vi "simple_subscriber_try.vi"() -> ()   [LabVIEW 2014]
panel:
  out "JSON字符串 2":string
  in  "停止":bool
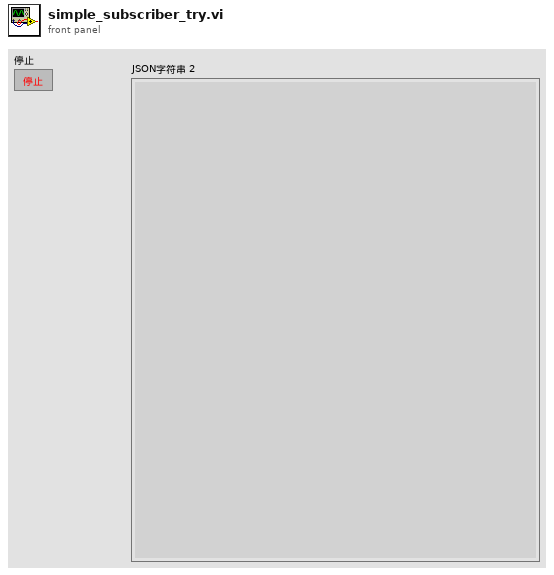
[diagram p1: front panel]
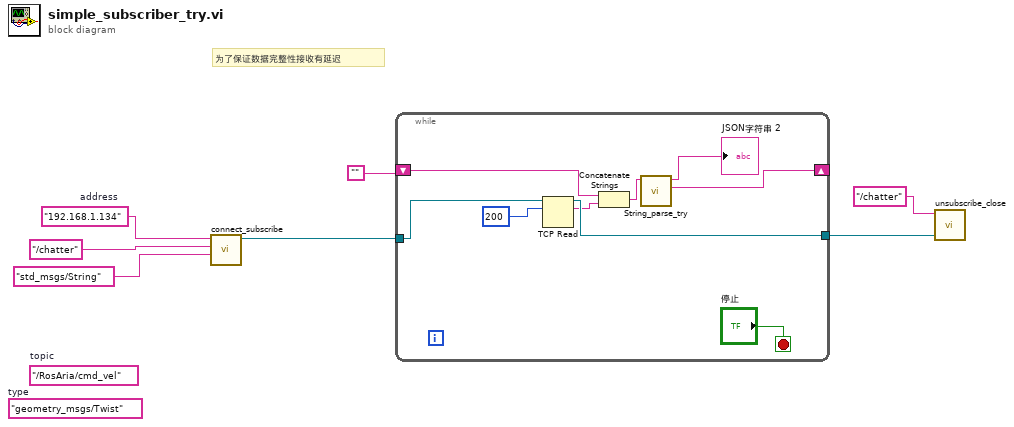
[diagram p0: block diagram]
diagram:
  (unwired) "geometry_msgs/Twist"  # type
  (unwired) "/RosAria/cmd_vel"  # topic
  w7 = "192.168.1.134"  # address
  # "为了保证数据完整性接收有延迟"
  n1 = call "connect_subscribe.vi"("type"="std_msgs/String", "topic"="/chatter", "address"=w7) -> ("连接ID输出"=w6:refnum<k5>)  [unwired: 7 in, 1 out]
  n2 = while {
    tunnel: [w16] -> w3
    tunnel: w6 -> [w13]
    shift-right: [w8] -> _
    shift-left: "" -> [w11]
    stop <- "停止" stop-if-true
    n3 = TCP Read(connection ID=w13, bytes to read=200 ("读取的字节")) -> (connection ID out=w16:refnum<k5>, data out=w12:string)  [unwired: 3 in, 1 out]
    n4 = Concatenate Strings(w11, w12) -> (w10:string)
    n5 = call "String_parse_try.vi"("字符串"=w10) -> ("剩余字符串"=w8:string, "data"=→"JSON字符串 2":string)  [unwired: 9 in]
  }
  n6 = call "unsubscribe_close.vi"("连接ID"=w3, "topic"="/chatter") -> ()  [unwired: 10 in]
